vi "PFI-28000-System_Start Daemon.vi"(0 "PFI-28000-System in":refnum<class "PFI-28000-System.lvclass">, 11 "error in (no error)":errorcluster) -> (4 "PFI-28000-System out":refnum<class "PFI-28000-System.lvclass">, 15 "error out":errorcluster)   [LabVIEW 2017, in "PFI-28000-System.lvclass"]
uses:
  PFI-28000-System.lvclass
  PFI-28000-System.lvclass/PFI-28000-System.ctl
  PFI-28000-System_Daemon.vi
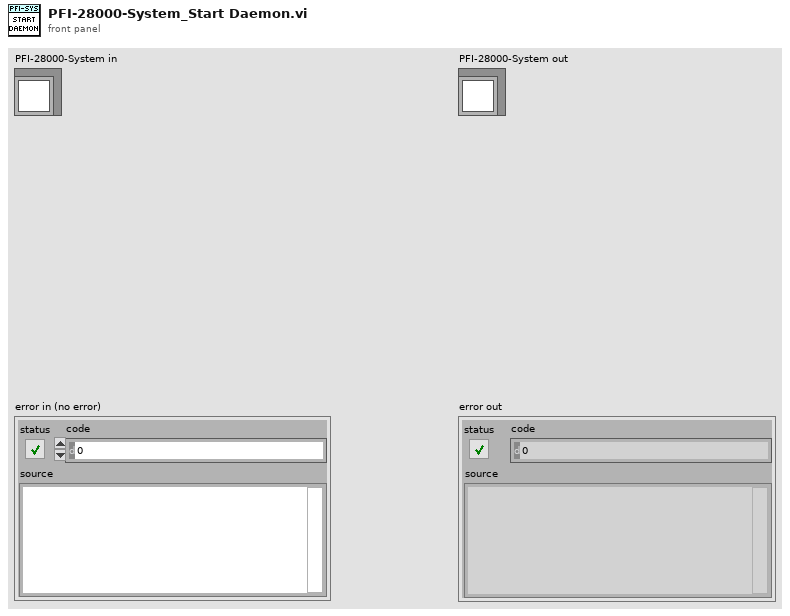
[diagram p1: front panel]
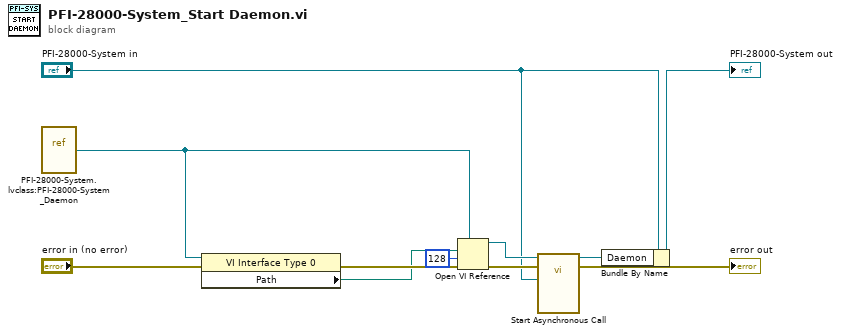
[diagram p0: block diagram]
diagram:
  n1 = vi-ref "PFI-28000-System.lvclass:PFI-28000-System_Daemon.vi"() -> (w10:refnum<vi>)
  n2 = property class="VI Interface Type 0"(reference=w10, error in="error in (no error)") -> (error out=w11:errorcluster, "Path"=w1:path)  [unwired: 1 out]
  n3 = Open VI Reference(type specifier VI Refnum (for type only)=w10, vi path=w1, options=128, error in (no error)=w11) -> (vi reference=w9:refnum<vi>, error out=w5:errorcluster)  [unwired: 2 in]
  n4 = call-by-ref "Start Asynchronous Call"(reference=w9, error in=w5, "PFI-28000-System"="PFI-28000-System in") -> (reference out=w2:refnum<vi>, error out=→"error out":errorcluster)  [unwired: 15 in]
  n5 = Bundle By Name(cluster="PFI-28000-System in", "Daemon"=w2) -> (→"PFI-28000-System out":refnum<class "PFI-28000-System.lvclass">)
